vi "CollectorWrapCheckInt.vi"(11 "Integer":i32) -> (3 "Changed?":bool)   [LabVIEW 2013]
doc: "Checks to see if the value of an integer has changed. If so, return true."
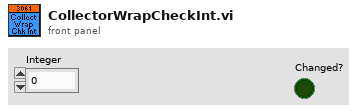
[diagram p1: front panel]
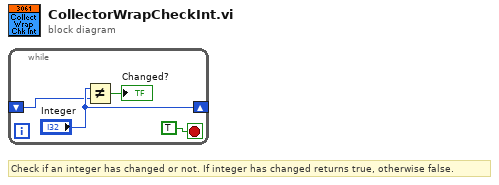
[diagram p0: block diagram]
diagram:
  # "Check if an integer has changed or not. If integer has changed returns true, otherwise false."
  n1 = while {
    shift-right: ["Integer"] -> _
    shift-left: _ -> [w2]
    stop <- TRUE stop-if-true
    n2 = Not Equal?(x="Integer", y=w2) -> (x != y?=→"Changed?":bool)
  }
